vi "write_node.vi"(8 "error in (no error)":errorcluster, 10 "Signals":dbl) -> (0 "error out":errorcluster)   [LabVIEW 2014]
panel:
  out "Filename Out 2":path caption="Filename Out"
  in  "True/False":bool
  # "Write Node\n\nwrites to excel file"
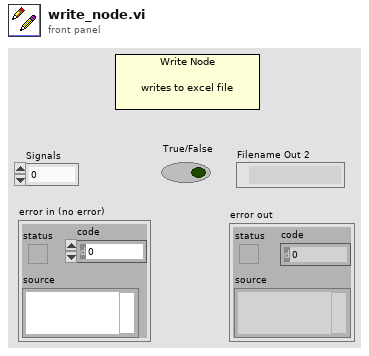
[diagram p1: front panel]
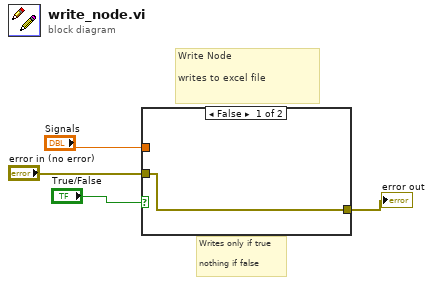
[diagram p0: block diagram]
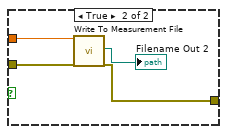
[diagram p2: hidden frame]
diagram:
  # "Writes only if true\n\nnothing if false"
  # "Write Node\n\nwrites to excel file"
  n1 = case shown="False" "True/False" {
    tunnel: "Signals" -> [_ w9]
    tunnel: "error in (no error)" -> [w5 w7]
    tunnel: [w5 w6] -> w1
    frame False {
    }
    frame True {
      n2 = call "Write To Measurement File"("Signals"=w9, "error in (no error)"=w7) -> ("Filename Out"=→"Filename Out 2":path, "error out"=w6:errorcluster)  [unwired: 15 in, 1 out]
    }
  }
  "error out" <- w1
